vi "DelayScanSetup.vi"(7 "Rep. Rate (Hz)":dbl=10.0 min=0.0 max=34.0, 10 "Start Position":dbl[](array[numeric]) min=0.0 max=34.0) -> (0 "BNC_Ctrl":bool, 1 "start/end points":cluster{dbl, dbl, dbl}[][](array[cluster]), 2 "Canceled":bool, 3 "DelayArray":dbl[](array[numeric]), 5 "ImageParameter":T1)   [LabVIEW 2013]
uses:
  ImagingMS/ImageConvPara.ctl
panel:
  in  "EndDelay":dbl=100.0 caption="End Delay (ps))" min=0.0 max=34.0
  in  "StartDelay":dbl caption="Start Delay (ps)" min=0.0 max=34.0
  in  "DelayStep":dbl=5.0 caption="Delay Step (ps)" min=0.0 max=34.0
  in  "ZeroDelayPos":dbl=8.016 caption="0 Delay (mm)" min=0.0 max=34.0
  in  "X StepWidth":dbl=0.025 min=0.0 max=34.0
  in  "LaserControl":bool=TRUE
  out "Estimated Time (min)":dbl min=0.0 max=34.0
  in  "Average/step":i32=10 min=0 max=34
  in  "Apply":bool
  in  "Cancel":bool
  in  "Run":bool
  out "XY Graph":cluster{dbl, dbl, "X StepWidth":dbl}[](graph)
  out "Y Size (mm)":dbl min=0.0 max=34.0
  out "X Size (mm)":dbl min=0.0 max=34.0
  out "Y Steps":i32=50 min=0 max=34
  in  "X Size":dbl=1.0 min=0.0 max=34.0
  in  "Y StepWidth":dbl=0.025 min=0.0 max=34.0
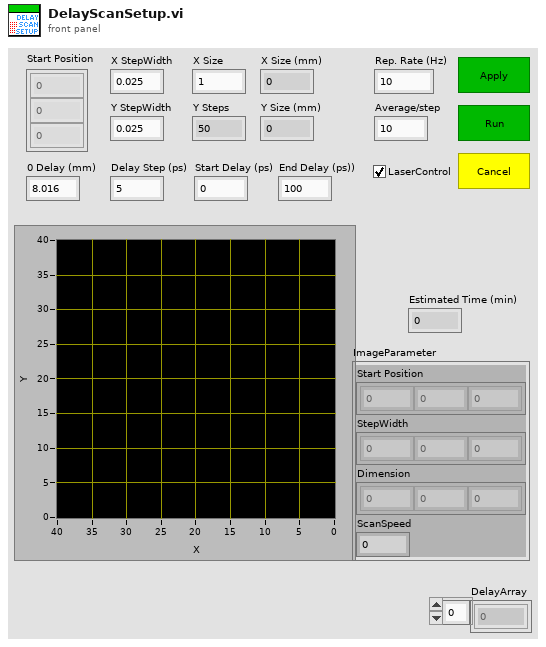
[diagram p1: front panel]
types:
  T1 = typedef "ImageConvPara.ctl" = cluster{"Start Position":dbl[], "StepWidth":dbl[], "Dimension":i32[], "ScanSpeed":dbl}
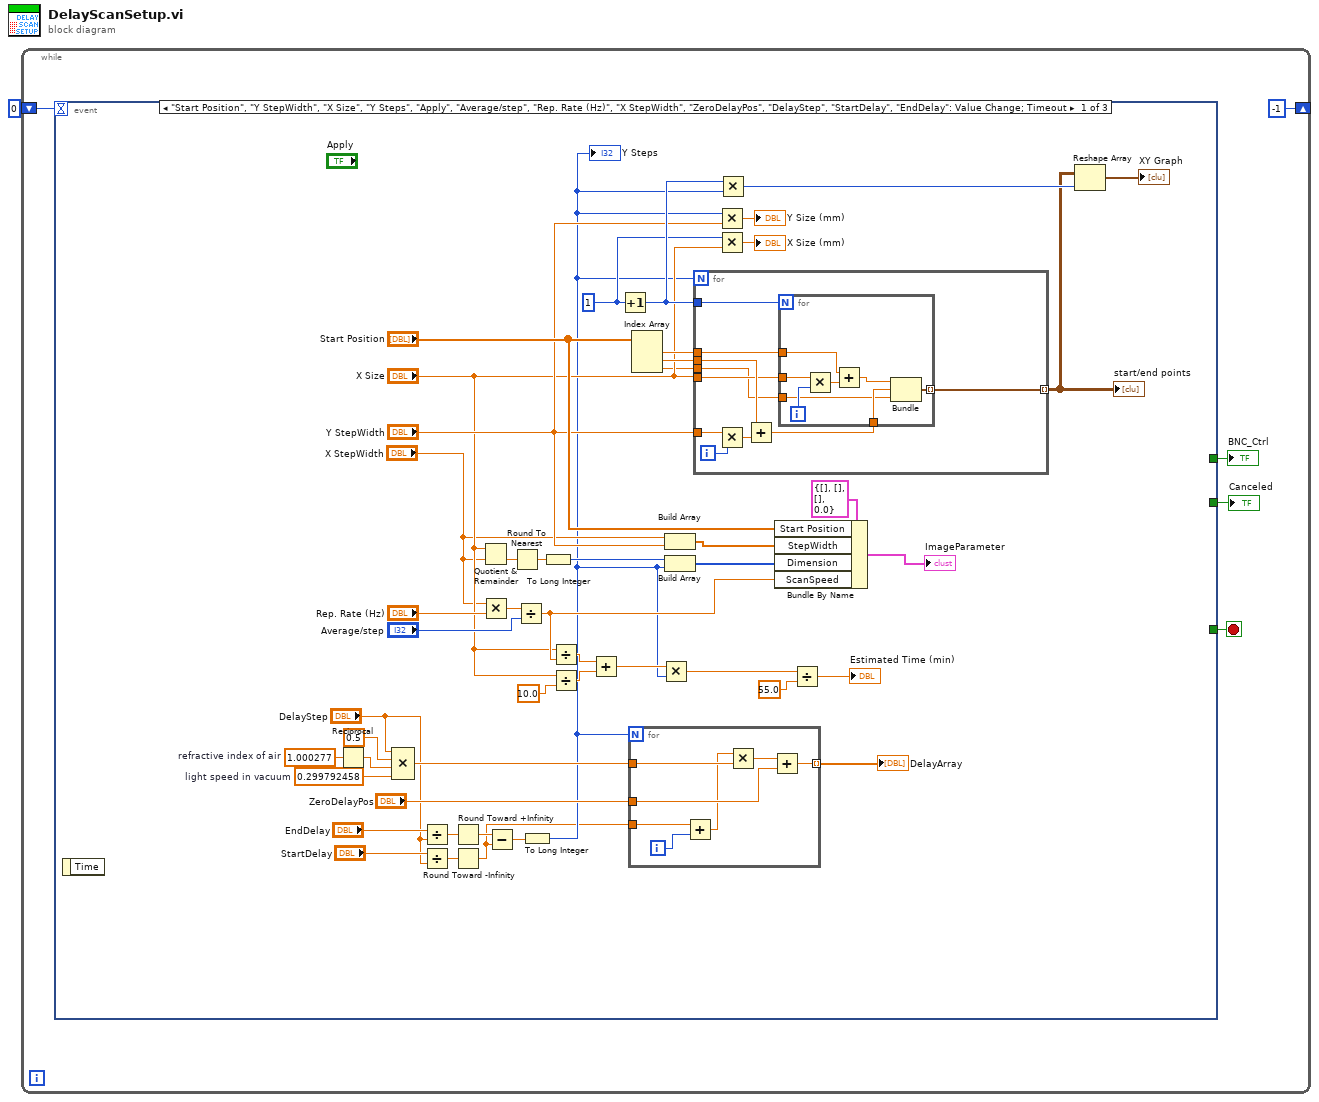
[diagram p0: block diagram]
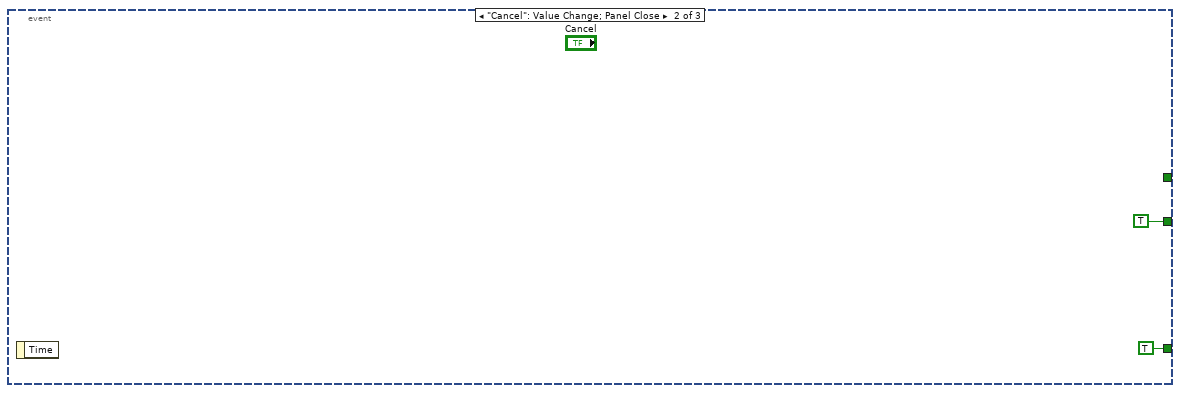
[diagram p2: hidden frame]
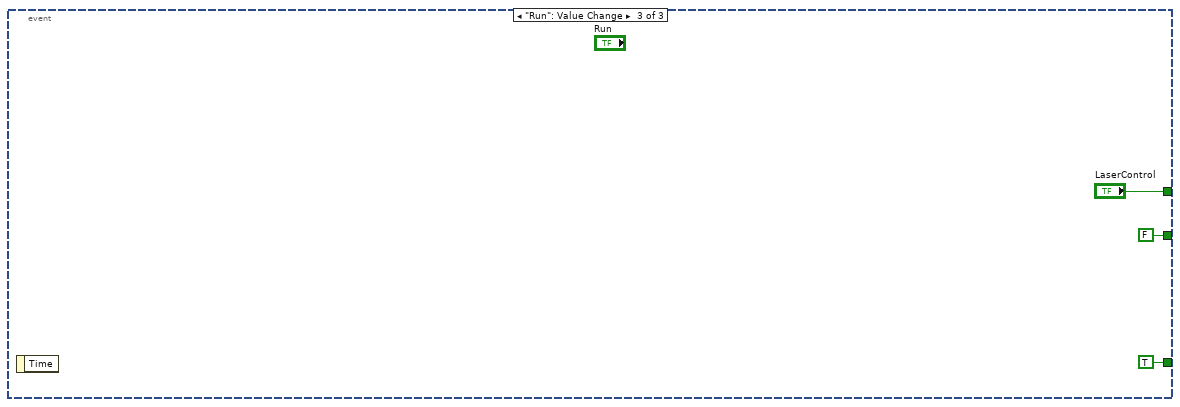
[diagram p3: hidden frame]
diagram:
  n1 = while {
    shift-right: [-1] -> _
    shift-left: 0 -> [w3]
    stop <- w6 stop-if-true
    n2 = event shown="[0] \"Start Position\", \"Y StepWidth\", \"X Size\", \"Y Steps\", \"Apply\", \"Average/step\", \"Rep. Rate (Hz)\", \"X StepWidth\", \"ZeroDelayPos\", \"DelayStep\", \"StartDelay\", \"EndDelay\": Value Change;  Timeout" {
      selector: _ -> [_ _ _]
      dyn-events: _ -> [_ _ _]
      timeout: w3 -> [_ _ _]
      tunnel: [_ TRUE TRUE] -> w6
      tunnel: [_ TRUE ("Canceled") FALSE ("Canceled")] -> w5
      tunnel: [_ _ "LaserControl"] -> w4
      event "Start Position", "Y StepWidth", "X Size", "Y Steps", "Apply", "Average/step", "Rep. Rate (Hz)", "X StepWidth", "ZeroDelayPos", "DelayStep", "StartDelay", "EndDelay": Value Change; Timeout {
        w20 = 0.299792458  # light speed in vacuum
        w21 = 1.000277  # refractive index of air
        w48 = 1
        n3 = event-data() -> ()  [unwired: 1 in, 1 out]
        n4 = Reciprocal(x=w21) -> (1/x=w7:dbl)
        n5 = Compound Arithmetic op=MULTIPLY("DelayStep", 0.5, w7, w20) -> (w18:dbl)
        n6 = Divide(x="EndDelay", y="DelayStep") -> (x/y=w14:dbl)
        n7 = Divide(x="StartDelay", y="DelayStep") -> (x/y=w13:dbl)
        n8 = Round Toward +Infinity(x=w14) -> (ceil(x): smallest int >= x=w12:dbl)
        n9 = Round Toward -Infinity(1:w13) -> (0:w8:dbl)
        n10 = Quotient & Remainder(x="X Size", y="X StepWidth") -> (floor(x/y)=w40:dbl)  [unwired: 1 out]
        n11 = Multiply(x="X StepWidth", y="Rep. Rate (Hz)") -> (x*y=w39:dbl)
        n12 = Subtract(x=w12, y=w8) -> (x-y=w10:dbl)
        n13 = Round To Nearest(number=w40) -> (nearest integer value=w24:dbl)
        n14 = Divide(x=w39, y="Average/step") -> (x/y=w35:dbl)
        n15 = To Long Integer(number=w10) -> (32bit integer=w9:i32)
        "Y Steps" <- w9
        n16 = To Long Integer(number=w24) -> (32bit integer=w25:i32)
        n17 = Divide(x="X Size", y=w35) -> (x/y=w33:dbl)
        n18 = Divide(x="X Size", y=10.0) -> (x/y=w32:dbl)
        n19 = Add(x=w33, y=w32) -> (x+y=w31:dbl)
        n20 = Increment(x=w48) -> (x+1=w49:i32)
        n21 = for {
          N: w9 -> [_]
          tunnel: w18 -> [w60]
          tunnel: "ZeroDelayPos" -> [w61]
          tunnel: w8 -> [w57]
          tunnel: [w55] -> w11 mode=indexing
          i -> [w58]
          n22 = Add(x=w57, y=w58) -> (x+y=w56:dbl)
          n23 = Multiply(x=w56, y=w60) -> (x*y=w59:dbl)
          n24 = Add(x=w59, y=w61) -> (x+y=w55:dbl)
        }
        "DelayArray" <- w11
        n25 = Index Array(array="Start Position") -> (element #1=w54:dbl, element #2=w53:dbl, element #3=w26:dbl)  [unwired: 3 in]
        n26 = Multiply(x=w31, y=w9) -> (x*y=w30:dbl)
        n27 = Build Array("X StepWidth", "Y StepWidth") -> (w43:dbl[])
        n28 = Build Array(w25, w9) -> (w42:i32[])
        n29 = for {
          N: w9 -> [_]
          tunnel: w53 -> [w66]
          tunnel: "Y StepWidth" -> [w62]
          tunnel: "X Size" -> [w65]
          tunnel: w49 -> [w68]
          tunnel: [w67] -> w46 mode=indexing
          tunnel: w26 -> [w63]
          tunnel: w54 -> [w64]
          i -> [w71]
          n30 = Multiply(x=w62, y=w71) -> (x*y=w70:dbl)
          n31 = Add(x=w66, y=w70) -> (x+y=w69:dbl)
          n32 = for {
            N: w68 -> [_]
            tunnel: w65 -> [w77]
            tunnel: w64 -> [w72]
            tunnel: w69 -> [w75]
            tunnel: [w76] -> w67 mode=indexing
            tunnel: w63 -> [w73]
            i -> [w78]
            n33 = Multiply(x=w77, y=w78) -> (x*y=w79:dbl)
            n34 = Add(x=w72, y=w79) -> (x+y=w74:dbl)
            n35 = Bundle(w74, w75, "X StepWidth"=w73) -> (w76:cluster{dbl, dbl, "X StepWidth":dbl})  [unwired: 1 in]
          }
        }
        "start/end points" <- w46
        n36 = Multiply(x=w9, y="Y StepWidth") -> (x*y=→"Y Size (mm)":dbl)
        n37 = Multiply(x=w48, y="X Size") -> (x*y=→"X Size (mm)":dbl)
        n38 = Multiply(x=w49, y=w9) -> (x*y=w50:i32)
        n39 = Bundle By Name(cluster=T1 {"Start Position"=[], "StepWidth"=[], "Dimension"=[], "ScanSpeed"=0.0} ("ImageParameter"), "Start Position"="Start Position", "StepWidth"=w43, "Dimension"=w42, "ScanSpeed"=w35) -> (→"ImageParameter":T1)
        n40 = Divide(x=w30, y=55.0) -> (x/y=→"Estimated Time (min)":dbl)
        n41 = Reshape Array(w46, w50) -> (→"XY Graph":cluster{dbl, dbl, "X StepWidth":dbl}[])
      }
      event "Cancel": Value Change; Panel Close {
        n42 = event-data() -> ()  [unwired: 1 in, 1 out]
      }
      event "Run": Value Change {
        n43 = event-data() -> ()  [unwired: 1 in, 1 out]
      }
    }
    "Canceled" <- w5
    "BNC_Ctrl" <- w4
  }
